vi "Actor Core.vi"(8 "error in":errorcluster, 11 "Active Station View Definition In":refnum<class "Active Option View Definition.lvclass">) -> (0 "error out":errorcluster, 3 "Actor out":refnum<class "Actor.lvclass">)   [LabVIEW 2019, in "Active Option View Definition.lvclass"]
doc: "(<B>Filename</B>: Actor Framework.lvlib:Actor.lvclass:Actor Core.vi)\n\nReceives messages to the actor, reacts to them, and initiates any error handling that may shut the actor down.\n\nDescendant classes may override this VI to append parallel tasks for the actor to complete while it handles messages. Overrides use the Call Parent Method node.\n\n<License>\nCopyright © 2017 Composed Systems, LLC | All rights reserved\nwww.composed.io\n\nAuthor: Ethan Stern <ethan.stern@composed.io>\n\nThis software is provided \"AS IS\" WITHOUT WARRANTIES, either express or implied, AND IS FOR EDUCATIONAL PURPOSES ONLY.\n</License>"
uses:
  <vilib>/gpm_packages/@cs/Car-wash/Source/Active Station View Definition/Active Station View Definition/Active Option View Definition.lvclass
  <vilib>/gpm_packages/@cs/mva-viewable/Source/IViewable/IViewable/IViewable.lvclass
  <vilib>/gpm_packages/@cs/mva-core/Source/IObserver/IObserver/IObserver.lvclass
  <vilib>/gpm_packages/@cs/Car-wash/Source/Active Station View Definition/Active Option View Definition Messages/Initialize Active Options Msg/Initialize Active Options Msg.lvclass
  <vilib>/gpm_packages/@cs/mva-core/Source/SubscriptionPolicy/BasicSubscription/BasicSubscription.lvclass
  C:/Program Files/National Instruments/LabVIEW 2019/vi.lib/gpm_packages/@cs/mva-viewable/Source/IViewable/IViewable/IViewable.lvclass
  C:/Program Files/National Instruments/LabVIEW 2019/vi.lib/gpm_packages/@cs/mva-core/Source/IObserver/IObserver/IObserver.lvclass
  C:/Program Files/National Instruments/LabVIEW 2019/vi.lib/gpm_packages/@cs/mva-core/Source/IMediator/ISubscriptionPolicy/ISubscriptionPolicy.lvclass
  C:/Program Files/National Instruments/LabVIEW 2019/vi.lib/gpm_packages/@cs/transport/Source/Concrete/ActorMessageTransport/Notification Msg/Notification Msg.lvclass
  <vilib>/ActorFramework/Actor/Actor.lvclass
panel:
  # "This is a definition view"
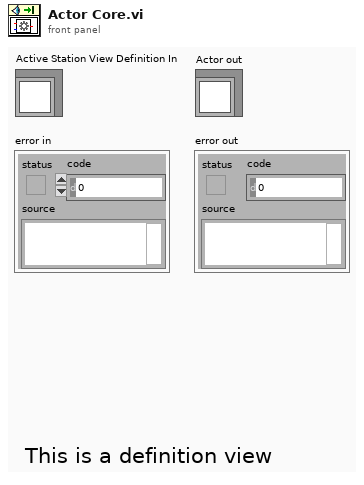
[diagram p1: front panel]
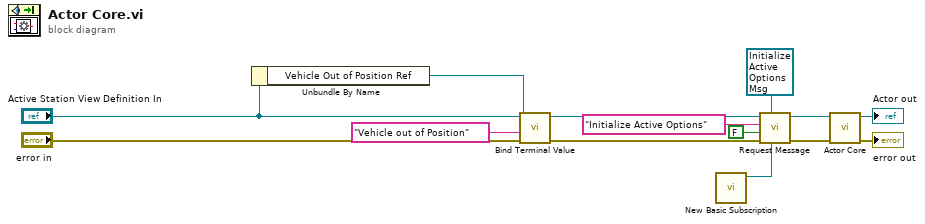
[diagram p0: block diagram]
diagram:
  n1 = Unbundle By Name("Active Station View Definition In") -> ("Vehicle Out of Position Ref"=w10:refnum<vi>)
  n2 = call <vilib>:"Bind Terminal Value.vi"("error in (no error)"="error in", "Datum Name (\"\"=Use Control Label)"="Vehicle out of Position" ("Datum Name (\"\"=Use Control Label)"), "Ctl Refnum"=w10, "IViewable in"="Active Station View Definition In") -> ("error out"=w6:errorcluster, "IViewable out"=w8:refnum<class "Active Option View Definition.lvclass">)  [unwired: 6 in]
  n3 = call <vilib>:"New Basic Subscription.vi"() -> ("BasicSubscription Out"=w1:refnum<class "BasicSubscription.lvclass">)  [unwired: 11 in]
  n4 = call <vilib>:"Request Message.vi"("Configured SubscriptionPolicy"=w1, "Desired Notification Msg"=refnum<class "Initialize Active Options Msg.lvclass"> refnum ("Initialize Active Options Msg.lvclass"), "error in (no error)"=w6, "Data Type"=FALSE, "Datum Name"="Initialize Active Options", "IObserver in"=w8) -> ("error out"=w5:errorcluster, "IObserver out"=w7:refnum<class "Active Option View Definition.lvclass">)  [unwired: 3 in, 1 out]
  n5 = call-parent "Actor Core.vi"("error in"=w5, "IViewable In"=w7) -> ("error out"=→"error out":errorcluster, "Actor out"=→"Actor out":refnum<class "Actor.lvclass">)  [unwired: 8 in]
